vi "Temporary_Cold_Wire_Spike_Replacer.vi"(2 "Data in":dbl[](array[numeric]), 3 "St Dev threshold":dbl=10.0) -> (0 "Data out":dbl[](array[numeric]), 1 "Points Replaced":i32)   [LabVIEW 2022 SP3]
uses:
  <vilib>/Analysis/baseanly.llb/Mean (DBL).vi
  Globals/Meas_global.vi
  Globals/Dynamic_call_global.ph.vi
  <vilib>/Analysis/NI_AALBase.lvlib
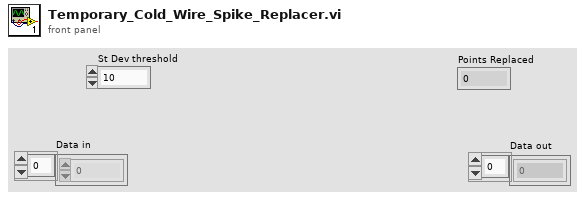
[diagram p1: front panel]
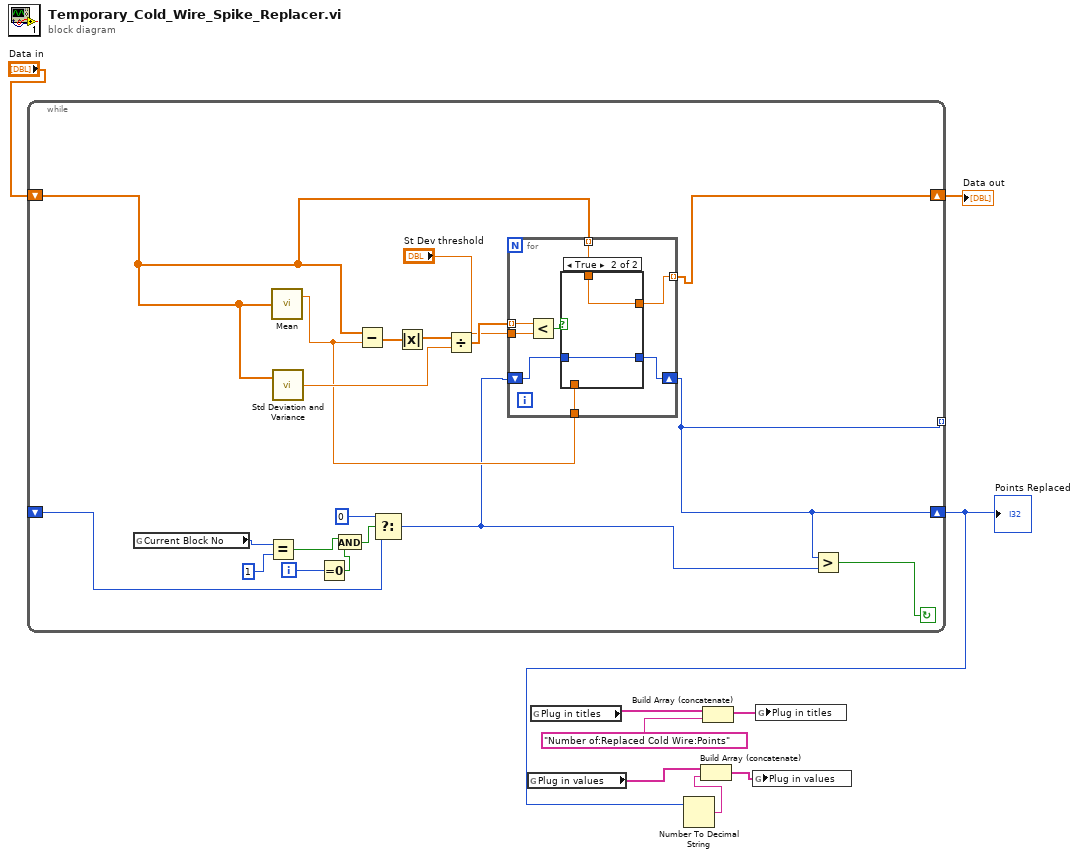
[diagram p0: block diagram]
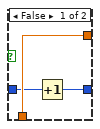
[diagram p2: hidden frame]
diagram:
  n1 = while {
    shift-right: [w10] -> w4
    shift-left: _ -> [w20]
    shift-right: [w18] -> w1
    shift-left: "Data in" -> [w19]
    tunnel: [w10] -> _ mode=indexing
    i -> [w17]
    stop <- w11 continue-if-true
    n2 = global read "Meas_global.vi" "Current Block No"() -> (w22:i32)
    n3 = Equal?(x=w22, y=1) -> (x = y?=w15:bool)
    n4 = call-poly <vilib>:"Mean.vi"("X"=w19) -> ("mean"=w23:dbl)  [unwired: 1 out]
    n5 = call <vilib>:"Std Deviation and Variance.vi"("X"=w19) -> ("standard deviation"=w26:dbl)  [unwired: 1 in, 2 out]
    n6 = Equal To 0?(x=w17) -> (x = 0?=w14:bool)
    n7 = And(x=w15, y=w14) -> (x .and. y?=w13:bool)
    n8 = Subtract(x=w19, y=w23) -> (x-y=w28:dbl[])
    n9 = Select(t=0, s=w13, f=w20) -> (s? t:f=w12:i32)
    n10 = Absolute Value(x=w28) -> (abs(x)=w27:dbl[])
    n11 = Divide(x=w27, y=w26) -> (x/y=w25:dbl[])
    n12 = for {
      tunnel: w25 -> [w35] mode=indexing
      tunnel: "St Dev threshold" -> [w36]
      tunnel: [w33] -> w18 mode=indexing
      tunnel: w19 -> [w34] mode=indexing
      tunnel: w23 -> [w32]
      shift-right: [w29] -> w10
      shift-left: w12 -> [w30]
      n13 = Less?(x=w35, y=w36) -> (x < y?=w31:bool)
      n14 = case shown="True" w31 {
        tunnel: w34 -> [_ w41]
        tunnel: [w39 w41] -> w33
        tunnel: w32 -> [w39 _]
        tunnel: w30 -> [w38 w40]
        tunnel: [w37 w40] -> w29
        frame False {
          n15 = Increment(x=w38) -> (x+1=w37:i32)
        }
        frame True {
        }
      }
    }
    n16 = Greater?(x=w10, y=w12) -> (0:w11:bool)
  }
  "Points Replaced" <- w4
  "Data out" <- w1
  n17 = global read "Dynamic_call_global.ph.vi" "Plug in values"() -> (w9:string[])
  n18 = global read "Dynamic_call_global.ph.vi" "Plug in titles"() -> (w8:string[])
  n19 = Number To Decimal String(number=w4) -> (decimal integer string=w3:string)  [unwired: 1 in]
  n20 = Build Array (concatenate)(w9, w3) -> (w7:string[])
  n21 = Build Array (concatenate)(w8, "Number of:Replaced Cold Wire:Points") -> (w6:string[])
  n22 = global write "Dynamic_call_global.ph.vi" "Plug in values"(w7) -> ()
  n23 = global write "Dynamic_call_global.ph.vi" "Plug in titles"(w6) -> ()
